vi "Read Interface object handle.vi"(8 "error in (no error)":errorcluster, 11 "DeviceNET in":refnum<class "DeviceNET.lvclass">) -> (0 "error out":errorcluster, 2 "ObjHandle":T1, 3 "DeviceNET out":refnum<class "DeviceNET.lvclass">)   [LabVIEW 2016, in "DeviceNET.lvclass"]
uses:
  DeviceNET.lvclass
  <vilib>/DeviceNet/VIAPI/subVIs/xobjhandle.ctl
  DeviceNET.lvclass/DeviceNET.ctl
  <vilib>/DeviceNet/DeviceNetLIB.lvlib
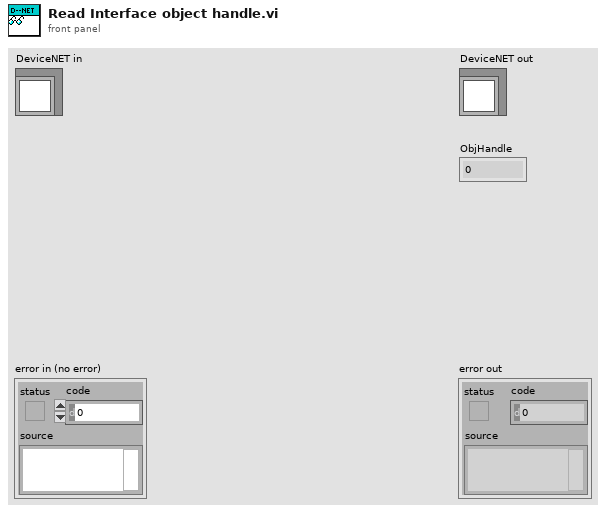
[diagram p1: front panel]
types:
  T1 = typedef "DeviceNetLIB.lvlib/xobjhandle.ctl" = u32
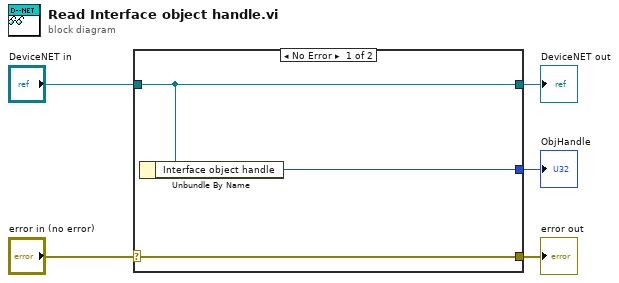
[diagram p0: block diagram]
diagram:
  n1 = case shown="No Error" "error in (no error)" {
    selector: "error in (no error)" -> [w8 w9]
    tunnel: [w8 w9] -> w4
    tunnel: [w7 w10] -> w2
    tunnel: "DeviceNET in" -> [w7 w10]
    tunnel: [w6 _] -> w1
    frame No Error {
      n2 = Unbundle By Name(w7) -> ("Interface object handle"=w6:T1)
    }
    frame Error {
    }
  }
  "error out" <- w4
  "DeviceNET out" <- w2
  "ObjHandle" <- w1
